vi "Turret Logic.vi"(0 "Turret Input":dbl, 1 "Turn Turret?":bool, 2 "Ticks":dbl, 3 "Timing":dbl) -> (5 "Value":dbl, 6 "Multiplier":dbl)   [LabVIEW 2019]
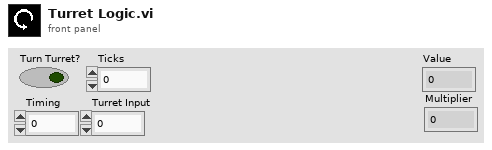
[diagram p1: front panel]
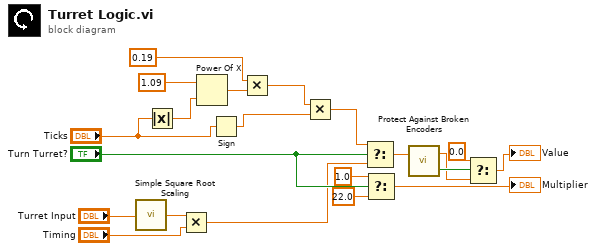
[diagram p0: block diagram]
diagram:
  n1 = call "Simple Square Root Scaling.vi"("Turret"="Turret Input") -> ("Scaled Value"=w18:dbl)
  n2 = Absolute Value(x="Ticks") -> (abs(x)=w5:dbl)
  n3 = Multiply(x=w18, y="Timing") -> (x*y=w6:dbl)
  n4 = Power Of X(1:w5, 2:1.09 ("y")) -> (0:w12:dbl)
  n5 = Sign(1:"Ticks") -> (0:w2:dbl)
  n6 = Multiply(x=0.19 ("Limelight Multiplier"), y=w12) -> (x*y=w3:dbl)
  n7 = Multiply(x=w3, y=w2) -> (x*y=w1:dbl)
  n8 = Select(t=w1, s="Turn Turret?", f=w6) -> (s? t:f=w11:dbl)
  n9 = Select(t=1.0, s="Turn Turret?", f=22.0 ("Multiplier")) -> (s? t:f=→"Multiplier":dbl)
  n10 = call "Protect Against Broken Encoders.vi"("Encoder Input"=w11) -> ("Broken"=w10:bool, "Output"=w7:dbl)  [unwired: 1 in]
  n11 = Select(t=0.0, s=w10, f=w7) -> (s? t:f=→"Value":dbl)
